vi "Frameremap_FBL.vi"(10 "Frame Origin (m)":cluster{"Xc":sgl, "Yc":sgl} {"Yc" format="%.2p"; "Xc" format="%.2p"}, 11 "Frame Size (m)":cluster{"Width":sgl, "Height":sgl} {"Height" format="%.2p"; "Width" format="%.2p"}) -> (0 "FH":dbl, 1 "FW":dbl, 2 "Z Origin":dbl, 3 "X Origin":dbl)   [LabVIEW 2019]
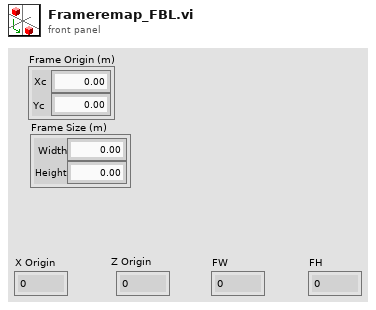
[diagram p1: front panel]
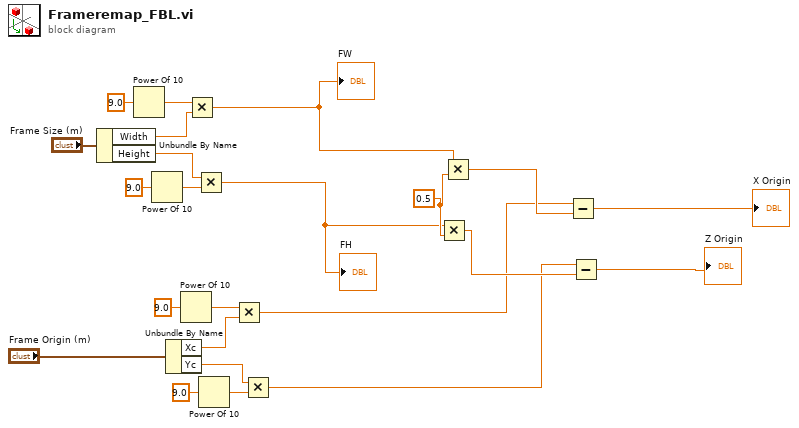
[diagram p0: block diagram]
diagram:
  w23 = 0.5 ("y")
  n1 = Unbundle By Name("Frame Size (m)") -> ("Width"=w15:sgl, "Height"=w12:sgl)
  n2 = Power Of 10(x=9.0) -> (10^x=w16:dbl)
  n3 = Power Of 10(x=9.0) -> (10^x=w14:dbl)
  n4 = Unbundle By Name("Frame Origin (m)") -> ("Xc"=w6:sgl, "Yc"=w5:sgl)
  n5 = Power Of 10(x=9.0) -> (10^x=w9:dbl)
  n6 = Multiply(x=w16, y=w15) -> (x*y=w2:dbl)
  "FW" <- w2
  n7 = Multiply(x=w12, y=w14) -> (x*y=w1:dbl)
  "FH" <- w1
  n8 = Power Of 10(x=9.0) -> (10^x=w8:dbl)
  n9 = Multiply(x=w9, y=w6) -> (x*y=w4:dbl)
  n10 = Multiply(x=w5, y=w8) -> (x*y=w3:dbl)
  n11 = Multiply(x=w1, y=w23) -> (x*y=w21:dbl)
  n12 = Multiply(x=w2, y=w23) -> (x*y=w22:dbl)
  n13 = Subtract(x=w4, y=w22) -> (x-y=→"X Origin":dbl)
  n14 = Subtract(x=w3, y=w21) -> (x-y=→"Z Origin":dbl)
